vi "Autptune_Points.vi"() -> ()   [LabVIEW 2018]
panel:
  in  "Commands":dbl[][](array[numeric])=[[8.0, 10.0, 0.0, 0.0, 0.0, 0.0, 0.0], [1.0, 0.0, -30.0, 30.0, 90.0, 60.0, 100.0], [17.0, 1.0, 0.0, 0.0, 0.0, 0.0, 0.0], [6.0, 0.5, 0.0, 0.0, 0.0, 0.0, 0.0], [1.0, 0.0, -30.0, 30.0, -90.0, 60.0, 270.0], [17.0, 2.0, 0.0, 0.0, 0.0, 0.0, 0.0], [6.0, 0.5, 0.0, 0.0, 0.0, 0.0, 0.0], [1.0, 0.0, -20.0, 20.0, 0.0, -90.0, 170.0], [17.0, 3.0, 0.0, 0.0, 0.0, 0.0, 0.0], [6.0, 0.5, 0.0, 0.0, 0.0, 0.0, 0.0], [1.0, 0.0, -20.0, 20.0, 0.0, -45.0, 190.0], [17.0, 4.0, 0.0, 0.0, 0.0, 0.0, 0.0], [6.0, 0.5, 0.0, 0.0, 0.0, 0.0, 0.0], [1.0, 0.0, -20.0, 20.0, 45.0, -45.0, 190.0], [17.0, 5.0, 0.0, 0.0, 0.0, 0.0, 0.0], [6.0, 0.5, 0.0, 0.0, 0.0, 0.0, 0.0], [1.0, -20.0, -30.0, 40.0, 45.0, 20.0, 270.0], [17.0, 6.0, 0.0, 0.0, 0.0, 0.0, 0.0], [6.0, 0.5, 0.0, 0.0, 0.0, 0.0, 0.0], [1.0, 20.0, -30.0, 40.0, 45.0, 20.0, 270.0], [17.0, 7.0, 0.0, 0.0, 0.0, 0.0, 0.0], [6.0, 0.5, 0.0, 0.0, 0.0, 0.0, 0.0], [1.0, 0.0, -30.0, 30.0, 0.0, 60.0, 180.0], [17.0, 8.0, 0.0, 0.0, 0.0, 0.0, 0.0], [8.0, 100.0, 0.0, 0.0, 0.0, 0.0, 0.0]]
  # "Commad\n6. Delay: subindex 1 is the pause in seconds.\n8. SetJointVel: subindex 1 is the percentage of maximum joint velocities, from 0.001 to 100%. (default: 25%)\n17. SetCheckpoint: subindex 1 in an integer number, ranging from 1 to 8,000."
  # "Colume 1 : Command\nColume 2 - 6 : Subindex"
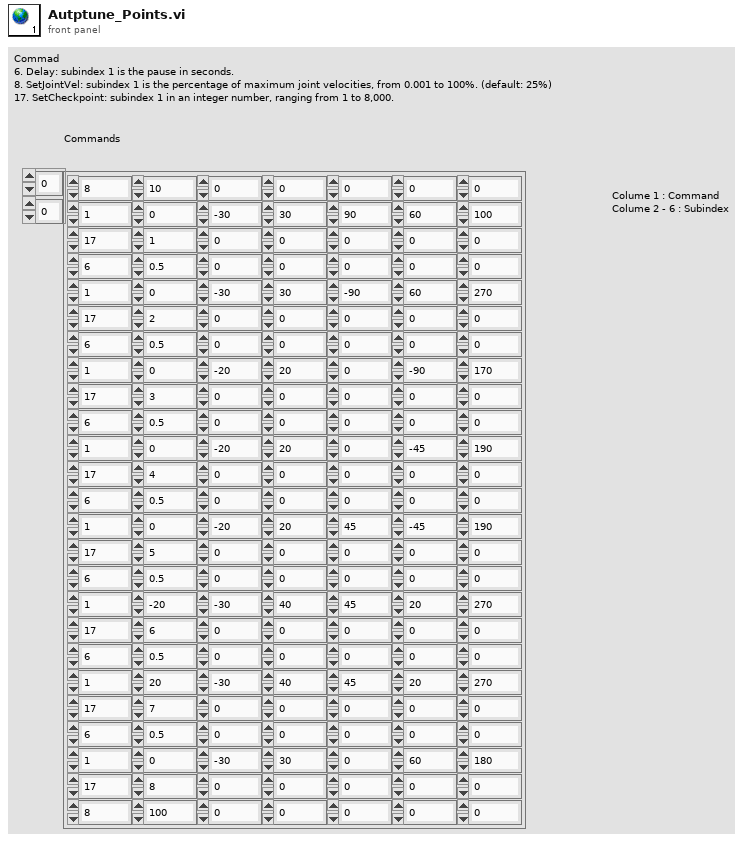
[diagram p1: front panel]
diagram:
